vi "Read Tektronix wfm header.vi"(8 "Error In":errorcluster, 11 "File Path":path) -> (0 "Error Out":errorcluster, 2 "Partial WFM header":T2 {"Bytes per point" format="%x"; "Byte order" format="%04x"}, 3 "WFM file ref out":T1={"refnum"=refnum, "byte order"=enum."little-endian", "Version"=0})   [LabVIEW 2015]
uses:
  WFM header.ctl
  WFM exp dimension.ctl
  WFM impl dimension.ctl
  WFM file ref.ctl
panel:
  out "offset (in bytes)":i64
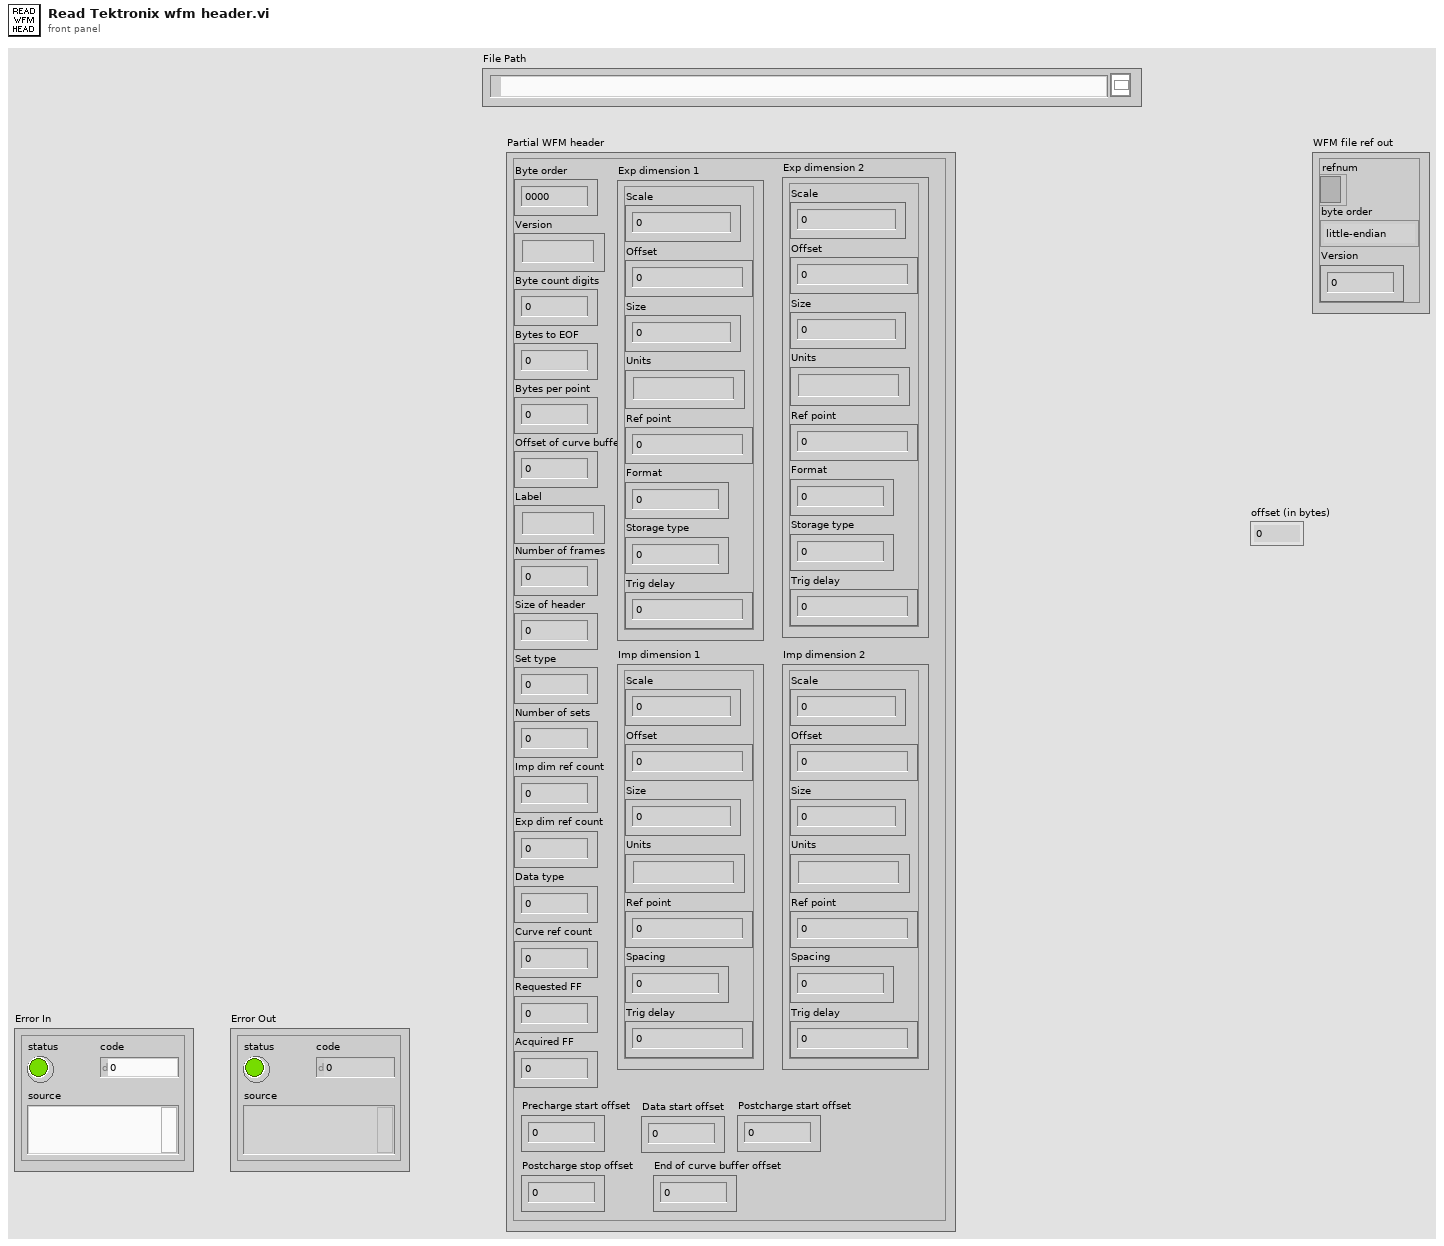
[diagram p1: front panel]
types:
  T1 = typedef "WFM file ref.ctl" = cluster{"refnum":refnum<file>, "byte order":enum16{"big-endian, network order", "native, host order", "little-endian"}, "Version":i32}
  T2 = typedef "WFM header.ctl" = cluster{"Byte order":u16, "Version":string, "Byte count digits":u8, "Bytes to EOF":i32, "Bytes per point":u8, "Offset of curve buffer":i32, "Label":string, "Number of frames":i32, "Size of header":u16, "Set type":i32, "Number of sets":i32, "Imp dim ref count":i32, "Exp dim ref count":i32, "Data type":i32, "Curve ref count":i32, "Requested FF":i32, "Acquired FF":i32, "Exp dimension 1":T3, "Exp dimension 2":T3, "Imp dimension 1":T4, "Imp dimension 2":T4, "Precharge start offset":i32, "Data start offset":i32, "Postcharge start offset":i32, "Postcharge stop offset":i32, "End of curve buffer offset":i32}
  T3 = typedef "WFM exp dimension.ctl" = cluster{"Scale":dbl, "Offset":dbl, "Size":i32, "Units":string, "Ref point":dbl, "Format":i32, "Storage type":i32, "Trig delay":dbl}
  T4 = typedef "WFM impl dimension.ctl" = cluster{"Scale":dbl, "Offset":dbl, "Size":i32, "Units":string, "Ref point":dbl, "Spacing":i32, "Trig delay":dbl}
  T5 = enum16{"big-endian, network order", "native, host order", "little-endian"}
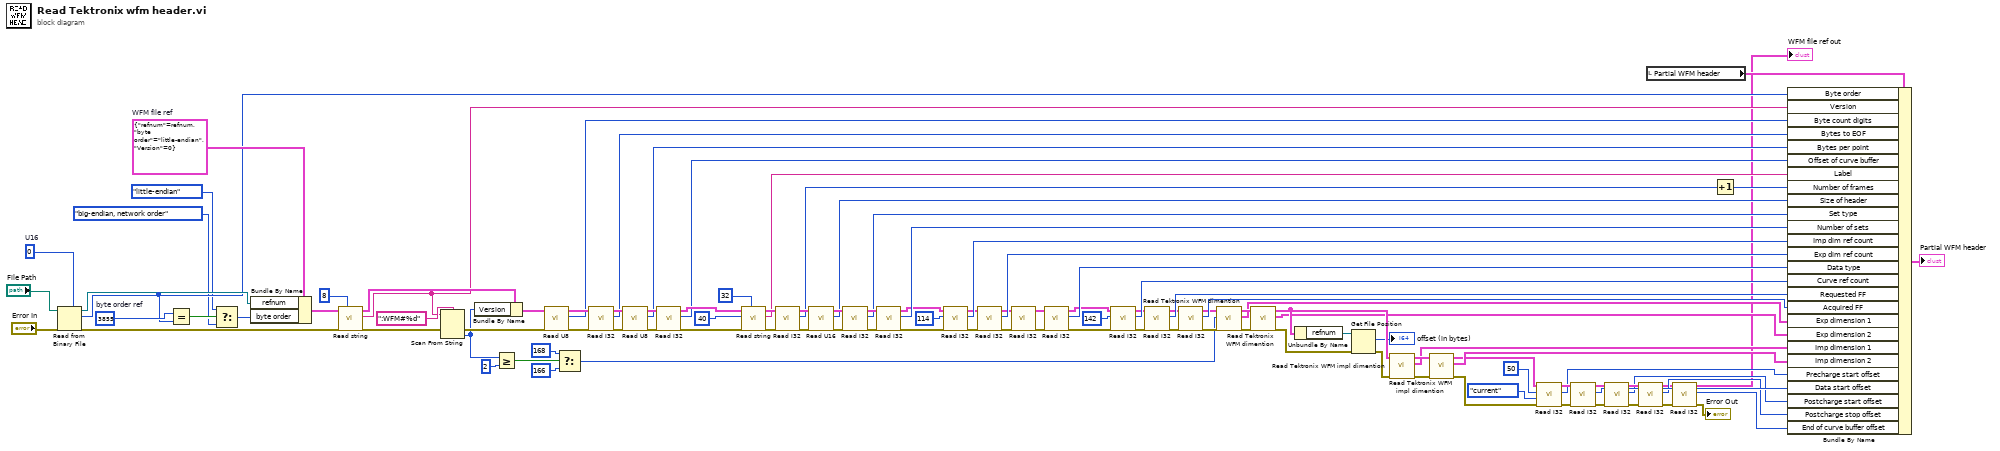
[diagram p0: block diagram]
diagram:
  w51 = u16 3855  # byte order ref
  w54 = T1 {"refnum"=refnum, "byte order"=enum."little-endian", "Version"=0}  # WFM file ref
  w112 = u16 0  # U16
  n1 = Read from Binary File(5:w112, 8:"Error In", 11:"File Path") -> (0:w100:errorcluster, 2:w50:u16, 3:w53:refnum<file>)  [unwired: 3 in, 1 out]
  n2 = Equal?(x=w51, y=w50) -> (x = y?=w49:bool)
  n3 = Select(t=T5."little-endian" ("byte order"), s=w49, f=T5."big-endian, network order" ("byte order")) -> (s? t:f=w46:T5)
  n4 = Bundle By Name(cluster=w54, "refnum"=w53, "byte order"=w46) -> (w52:T1)
  n5 = call "Read string.vi"("count (1)"=8, "Error In"=w100, "WFM file ref"=w52) -> ("Error Out"=w45:errorcluster, "data"=w42:string, "WFM file ref out"=w99:T1)  [unwired: 6 in]
  n6 = Scan From String(format string=":WFM#%d", input string=w42, error in=w45) -> (error out=w43:errorcluster, output 1=w33:i32)  [unwired: 2 in, 2 out]
  n7 = Bundle By Name(cluster=w99, "Version"=w33) -> (w34:T1)
  n8 = Greater Or Equal?(x=w33, y=2) -> (x >= y?=w39:bool)
  n9 = call "Read U8.vi"("Error In"=w43, "WFM file ref"=w34) -> ("Error Out"=w103:errorcluster, "data"=w91:u8, "WFM file ref out"=w102:T1)  [unwired: 7 in]
  n10 = Select(t=i64 168 ("offset (in bytes) (0)"), s=w39, f=i64 166 ("offset (in bytes) (0)")) -> (s? t:f=w35:i64)
  n11 = call "Read I32.vi"("Error In"=w103, "WFM file ref"=w102) -> ("Error Out"=w106:errorcluster, "data"=w90:i32, "WFM file ref out"=w107:T1)  [unwired: 7 in]
  n12 = call "Read U8.vi"("Error In"=w106, "WFM file ref"=w107) -> ("Error Out"=w104:errorcluster, "data"=w89:u8, "WFM file ref out"=w105:T1)  [unwired: 7 in]
  n13 = call "Read I32.vi"("Error In"=w104, "WFM file ref"=w105) -> ("Error Out"=w110:errorcluster, "data"=w88:i32, "WFM file ref out"=w109:T1)  [unwired: 7 in]
  n14 = call "Read string.vi"("count (1)"=32, "Error In"=w110, "offset (in bytes) (0)"=i64 40, "WFM file ref"=w109) -> ("Error Out"=w81:errorcluster, "data"=w87:string, "WFM file ref out"=w98:T1)  [unwired: 5 in]
  n15 = call "Read I32.vi"("Error In"=w81, "WFM file ref"=w98) -> ("Error Out"=w94:errorcluster, "data"=w83:i32, "WFM file ref out"=w97:T1)  [unwired: 7 in]
  n16 = call "Read U16.vi"("Error In"=w94, "WFM file ref"=w97) -> ("Error Out"=w93:errorcluster, "data"=w82:u16, "WFM file ref out"=w96:T1)  [unwired: 7 in]
  n17 = call "Read I32.vi"("Error In"=w93, "WFM file ref"=w96) -> ("Error Out"=w92:errorcluster, "data"=w85:i32, "WFM file ref out"=w95:T1)  [unwired: 7 in]
  n18 = call "Read I32.vi"("Error In"=w92, "WFM file ref"=w95) -> ("Error Out"=w77:errorcluster, "data"=w84:i32, "WFM file ref out"=w78:T1)  [unwired: 7 in]
  n19 = call "Read I32.vi"("Error In"=w77, "offset (in bytes) (0)"=i64 114, "WFM file ref"=w78) -> ("Error Out"=w74:errorcluster, "data"=w75:i32, "WFM file ref out"=w73:T1)  [unwired: 6 in]
  n20 = call "Read I32.vi"("Error In"=w74, "WFM file ref"=w73) -> ("Error Out"=w70:errorcluster, "data"=w72:i32, "WFM file ref out"=w71:T1)  [unwired: 7 in]
  n21 = call "Read I32.vi"("Error In"=w70, "WFM file ref"=w71) -> ("Error Out"=w68:errorcluster, "WFM file ref out"=w69:T1)  [unwired: 7 in, 1 out]
  n22 = call "Read I32.vi"("Error In"=w68, "WFM file ref"=w69) -> ("Error Out"=w66:errorcluster, "data"=w67:i32, "WFM file ref out"=w65:T1)  [unwired: 7 in]
  n23 = call "Read I32.vi"("Error In"=w66, "offset (in bytes) (0)"=i64 142, "WFM file ref"=w65) -> ("Error Out"=w61:errorcluster, "data"=w63:i32, "WFM file ref out"=w62:T1)  [unwired: 6 in]
  n24 = call "Read I32.vi"("Error In"=w61, "WFM file ref"=w62) -> ("Error Out"=w59:errorcluster, "data"=w60:i32, "WFM file ref out"=w58:T1)  [unwired: 7 in]
  n25 = call "Read I32.vi"("Error In"=w59, "WFM file ref"=w58) -> ("Error Out"=w55:errorcluster, "data"=w57:i32, "WFM file ref out"=w56:T1)  [unwired: 7 in]
  n26 = call "Read Tektronix WFM dimention.vi"("Error In"=w55, "offset (in bytes) (0)"=w35, "WFM file ref"=w56) -> ("Error Out"=w37:errorcluster, "Dimension"=w23:T3, "WFM file ref out"=w36:T1)  [unwired: 6 in]
  n27 = call "Read Tektronix WFM dimention.vi"("Error In"=w37, "WFM file ref"=w36) -> ("Error Out"=w31:errorcluster, "Dimension"=w22:T3, "WFM file ref out"=w32:T1)  [unwired: 7 in]
  n28 = Unbundle By Name(w32) -> ("refnum"=w29:refnum<file>)
  n29 = Get File Position(4:w31, 7:w29) -> (0:w30:errorcluster, 2:→"offset (in bytes)":i64)  [unwired: 1 out]
  n30 = call "Read Tektronix WFM impl dimention.vi"("Error In"=w30, "WFM file ref"=w32) -> ("Error Out"=w27:errorcluster, "Dimension"=w21:T4, "WFM file ref out"=w26:T1)  [unwired: 7 in]
  n31 = call "Read Tektronix WFM impl dimention.vi"("Error In"=w27, "WFM file ref"=w26) -> ("Error Out"=w18:errorcluster, "Dimension"=w20:T4, "WFM file ref out"=w19:T1)  [unwired: 7 in]
  n32 = call "Read I32.vi"("Error In"=w18, "from (0:start)"=enum16{"start", "end", "current"}."current", "offset (in bytes) (0)"=i64 50, "WFM file ref"=w19) -> ("Error Out"=w12:errorcluster, "data"=w9:i32, "WFM file ref out"=w13:T1)  [unwired: 5 in]
  n33 = call "Read I32.vi"("Error In"=w12, "WFM file ref"=w13) -> ("Error Out"=w14:errorcluster, "data"=w8:i32, "WFM file ref out"=w15:T1)  [unwired: 7 in]
  n34 = call "Read I32.vi"("Error In"=w14, "WFM file ref"=w15) -> ("Error Out"=w17:errorcluster, "data"=w7:i32, "WFM file ref out"=w16:T1)  [unwired: 7 in]
  n35 = call "Read I32.vi"("Error In"=w17, "WFM file ref"=w16) -> ("Error Out"=w5:errorcluster, "data"=w6:i32, "WFM file ref out"=w4:T1)  [unwired: 7 in]
  n36 = local read "Partial WFM header"() -> (w25:T2)
  n37 = call "Read I32.vi"("Error In"=w5, "WFM file ref"=w4) -> ("Error Out"=→"Error Out":errorcluster, "data"=w1:i32, "WFM file ref out"=→"WFM file ref out":T1)  [unwired: 7 in]
  n38 = Increment(x=w83) -> (x+1=w86:i32)
  n39 = Bundle By Name(cluster=w25, "Byte order"=w50, "Version"=w42, "Byte count digits"=w91, "Bytes to EOF"=w90, "Bytes per point"=w89, "Offset of curve buffer"=w88, "Label"=w87, "Number of frames"=w86, "Size of header"=w82, "Set type"=w85, "Number of sets"=w84, "Imp dim ref count"=w75, "Exp dim ref count"=w72, "Data type"=w67, "Curve ref count"=w63, "Requested FF"=w60, "Acquired FF"=w57, "Exp dimension 1"=w23, "Exp dimension 2"=w22, "Imp dimension 1"=w21, "Imp dimension 2"=w20, "Precharge start offset"=w9, "Data start offset"=w8, "Postcharge start offset"=w7, "Postcharge stop offset"=w6, "End of curve buffer offset"=w1) -> (→"Partial WFM header":T2)
